vi "Export Frame Data.vi"(8 "error in (no error)":errorcluster, 10 "File Format":string, 11 "FE FF Frame in":refnum<class "FE FF Frame.lvclass">) -> (0 "error out":errorcluster, 3 "FE FF Frame out":refnum<class "FE FF Frame.lvclass">)   [LabVIEW 2023, in "Data Analysis.lvlib" / "FE FF Frame.lvlib" / "FE FF Frame.lvclass"]
uses:
  FE FF Frame.lvclass
  FE FF Frame.lvclass/FE FF Frame.ctl
  <vilib>/Utility/file.llb/Write Delimited Spreadsheet (string).vi
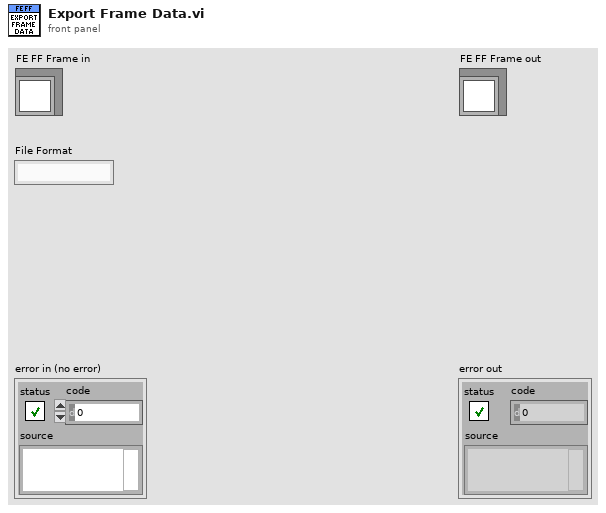
[diagram p1: front panel]
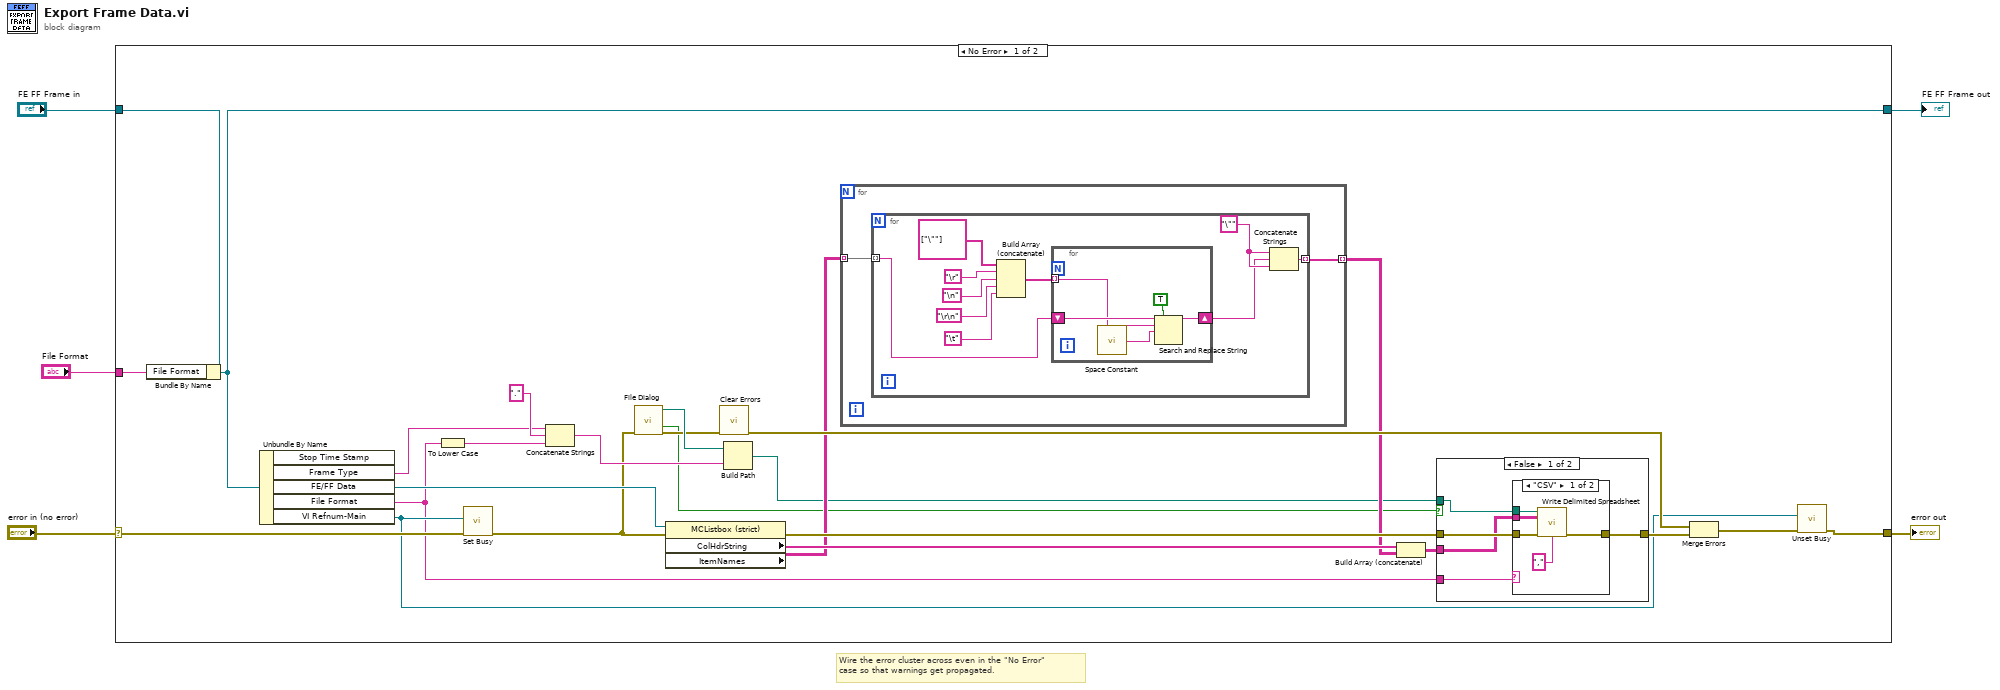
[diagram p0: block diagram]
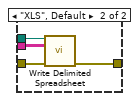
[diagram p2: hidden frame]
diagram:
  # "Wire the error cluster across even in the \"No Error\"\ncase so that warnings get propagated."
  n1 = case shown="No Error" "error in (no error)" {
    selector: "error in (no error)" -> [w22 w64]
    tunnel: [w19 w64] -> w4
    tunnel: [w21 w63] -> w2
    tunnel: "FE FF Frame in" -> [w24 w63]
    tunnel: "File Format" -> [w23 _]
    frame No Error {
      n2 = Bundle By Name(cluster=w24, "File Format"=w23) -> (w21:refnum<class "FE FF Frame.lvclass">)
      n3 = Unbundle By Name(w21) -> ("Frame Type"=w11:string, "FE/FF Data"=w27:refnum<vi>, "File Format"=w10:string, "VI Refnum-Main"=w18:refnum<vi>)  [unwired: 1 out]
      n4 = To Lower Case(string=w10) -> (all lower case string=w13:string)
      n5 = call <vilib>:"Set Busy.vi"("error in (no error)"=w22, "VI reference (current VI)"=w18) -> ("error out"=w9:errorcluster)  [unwired: 8 in, 1 out]
      n6 = Concatenate Strings(w11, "." ("pattern (all files)"), w13) -> (w12:string)
      n7 = call "File Dialog"("error in"=w9) -> ("selected path"=w15:path, "cancelled"=w6:bool, "error out"=w8:errorcluster)  [unwired: 11 in, 1 out]
      n8 = property class="MCListbox (strict)"(reference=w27, error in=w9) -> (error out=w30:errorcluster, "ColHdrString"=w28:string[], "ItemNames"=w17:string[][])  [unwired: 1 out]
      n9 = call <vilib>:"Clear Errors.vi"("error in (no error)"=w8) -> ("error out"=w25:errorcluster)  [unwired: 5 in, 1 out]
      n10 = Build Path(base path=w15, name or relative path=w12) -> (appended path=w7:path)
      n11 = for {
        tunnel: w17 -> [w32] mode=indexing
        tunnel: [w31] -> w16 mode=indexing
        n12 = for {
          tunnel: w32 -> [w34] mode=indexing
          tunnel: [w41] -> w31 mode=indexing
          w42 = "\""
          n13 = Build Array (concatenate)(string[] ["\""], "\r", "\n", "\r\n", "\t") -> (w40:string[])
          n14 = for {
            tunnel: w40 -> [w44] mode=indexing
            shift-right: [w45] -> w33
            shift-left: w34 -> [w46]
            n15 = call <vilib>:"Space Constant.vi"() -> ("String"=w43:string)
            n16 = Search and Replace String(replace all?=TRUE ("replace all? (F)"), input string=w46, search string=w44, replace string=w43) -> (result string=w45:string)  [unwired: 4 in, 3 out]
          }
          n17 = Concatenate Strings(w42, w33, w42) -> (w41:string)
        }
      }
      n18 = Build Array (concatenate)(w28, w16) -> (w29:string[][])
      n19 = case shown="False" w6 {
        tunnel: w30 -> [w52 w62]
        tunnel: [w51 w62] -> w26
        tunnel: w29 -> [w50 _]
        tunnel: w7 -> [w49 _]
        tunnel: w10 -> [w48 _]
        frame False {
          n20 = case shown="\"CSV\"" w48 {
            tunnel: w52 -> [w57 w61]
            tunnel: [w56 w60] -> w51
            tunnel: w50 -> [w55 w59]
            tunnel: w49 -> [w54 w58]
            frame "CSV" {
              n21 = call-poly <vilib>:"Write Delimited Spreadsheet.vi"("file path (dialog if empty)"=w54, "2D data"=w55, "error in (no error)"=w57, "delimiter (\\t)"="," ("delimiter (\\t)")) -> ("error out"=w56:errorcluster)  [unwired: 10 in, 1 out]
            }
            frame "XLS", Default {
              n22 = call-poly <vilib>:"Write Delimited Spreadsheet.vi"("file path (dialog if empty)"=w58, "2D data"=w59, "error in (no error)"=w61) -> ("error out"=w60:errorcluster)  [unwired: 11 in, 1 out]
            }
          }
        }
        frame True {
        }
      }
      n23 = Merge Errors(w25, w26) -> (w20:errorcluster)
      n24 = call <vilib>:"Unset Busy.vi"("error in (no error)"=w20, "VI reference (current VI)"=w18) -> ("error out"=w19:errorcluster)  [unwired: 9 in]
    }
    frame Error {
    }
  }
  "error out" <- w4
  "FE FF Frame out" <- w2
